vi "mySignInterpreter.vi"() -> ()   [LabVIEW 2017]
uses:
  LeapMotion/TypeDefs/SelectSign.ctl
  LeapMotion/TypeDefs/StateSelector.ctl
  LeapMotion/TypeDefs/AppData.ctl
  MachineLearning/TypeDefs/Label Setting.ctl
  C:/Users/Sara/Documents/GitHub/LEAP-sign-language/LEAP-sign-language/LeapMotion/Dynamic Libraries/LeapCSharp.NET4.5.dll
  LeapMotion/Dynamic Libraries/LeapCSharp.NET4.5.dll
  LeapMotion/LeapMotion.lvlib
  MachineLearning/MachineLearning.lvlib
panel:
  out "Hand count":i32
  in  "Clear text":bool
  in  "Interpret hand sign":bool
  out "Interpreted text":string
  in  "Tab Control":T1(tab)
  out "Real-time plot":cluster{sgl[], sgl[]}[](graph)
  out "Correct interpretations":i32
  out "Number of tries":i32
  out "feature trend":dbl[][](graph)
  out "predicted result":i32[][](graph)
  in  "Error In":errorcluster
  out "Error out":errorcluster
  in  "Trained ML model":path=path "C:/Users/Sara/Documents/GitHub/LEAP-sign-language/LEAP-sign-language/MachineLearning/SubVIs/Models/ASL-ABCD.json"
  out "Accuracy":dbl
  out "Detected sign":T2
  out "Logging in":i32
  in  "Delay":i32=3
  in  "Train model":bool
  out "Points to log":i32
  in  "Start logging":bool
  in  "Write header":bool
  in  "Points/sign":i32=100
  out "feature trend":dbl[][](graph)
  in  "Hand sign":T2
  in  "Stop Program":bool
  out "LEAP connected?":bool
  # "1"
  # "2"
  # "3"
  # "Logging sequence options"
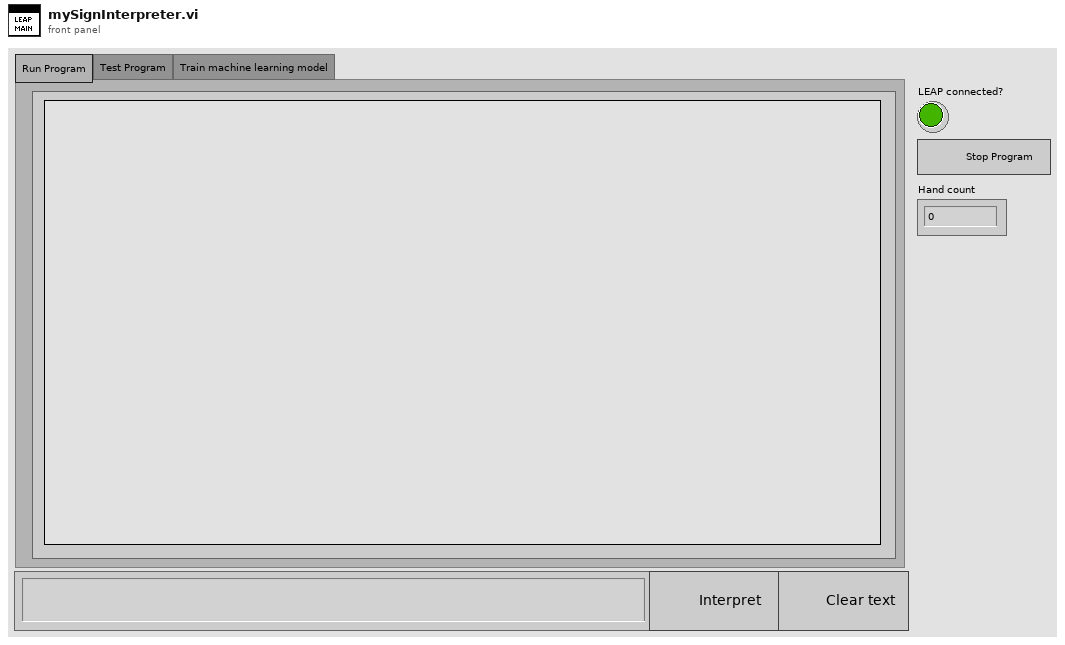
[diagram p1: front panel]
types:
  T1 = enum32{"Run Program", "Test Program", "Train machine learning model"}
  T2 = typedef "LeapMotion.lvlib/SelectSign.ctl" = enum16{"A", "B", "C", "D", "E", "F", "G", "H", "I", "J", "K", "L", "M", "N", "O", "P", "Q", "R", "S", "T", "U", "V", "W", "X", "Y", "Z"}
  T3 = typedef "LeapMotion.lvlib/AppData.ctl" = cluster{"File path":path, "LEAP":refnum<k24>}
  T4 = typedef "LeapMotion.lvlib/StateSelector.ctl" = enum16{"Initialize", "Display", "Write Header", "Logging", "Log gesture", "Train model", "Classify", "Stop"}
  T5 = typedef "MachineLearning.lvlib/Label Setting.ctl" = cluster{"with label column?":bool, "label column index":i32}
  T6 = typedef "LeapMotion.lvlib/LEAPframe.ctl" = cluster{"Id":i64, "Timestamp":i64, "CurrentFramesPerSecond":sgl, "Hands":T7[]}
  T7 = typedef "LeapMotion.lvlib/LEAPhand.ctl" = cluster{"IsLeft":bool, "IsRight":bool, "Id":i32, "FrameId":i64, "Confidence":sgl, "TimeVisible":sgl, "Arm":T8, "PalmPosition":T9, "Fingers":T10[]}
  T8 = typedef "LeapMotion.lvlib/LEAParm.ctl" = cluster{"WristXYZ":sgl[], "CenterXYZ":sgl[], "ElbowXYZ":sgl[]}
  T9 = typedef "LeapMotion.lvlib/LEAPvector.ctl" = cluster{"Pitch":sgl, "Yaw":sgl, "Roll":sgl, "Magnitude":sgl, "XYZ":sgl[]}
  T10 = typedef "LeapMotion.lvlib/LEAPfinger.ctl" = cluster{"IsExtended":bool, "Id":i32, "Type":i32, "HandId":i32, "Length":sgl, "Width":sgl, "TimeVisible":sgl, "TipPosition":T9, "TipVelocity":T9, "Bones":T11[]}
  T11 = typedef "LeapMotion.lvlib/LEAPbone.ctl" = cluster{"Type":i32, "Width":sgl, "Length":sgl, "Center":T9, "Direction":T9, "NextJoint":T9, "PrevJoint":T9}
  T12 = enum16{"SVM", "Neural Network", "Logistic Regression"}
  T13 = cluster{"accuracy":dbl, "precision":dbl, "recall":dbl, "f1 score":dbl}
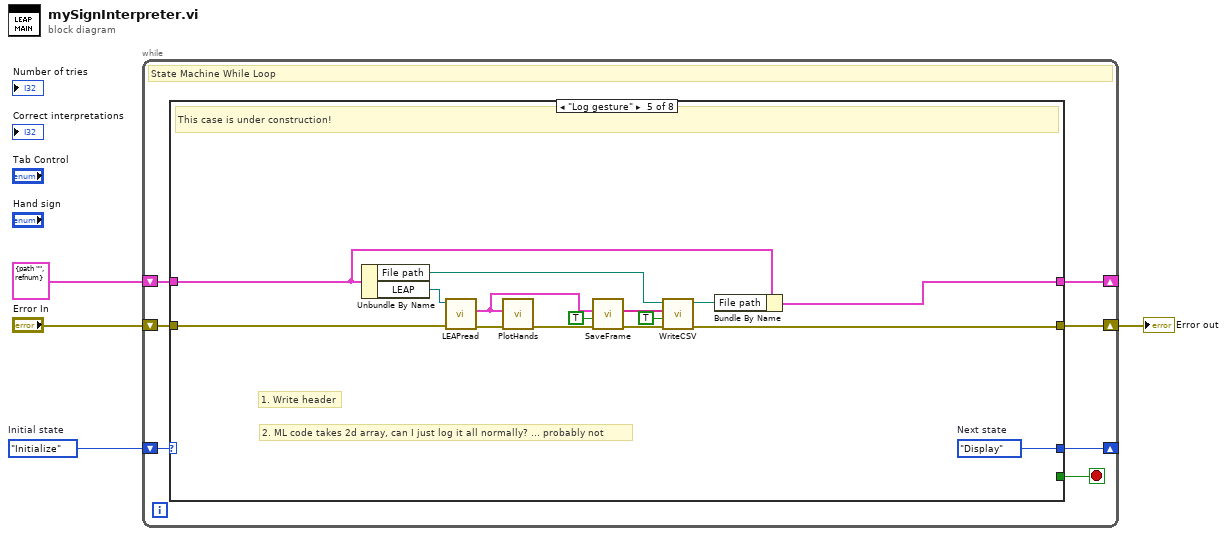
[diagram p0: block diagram]
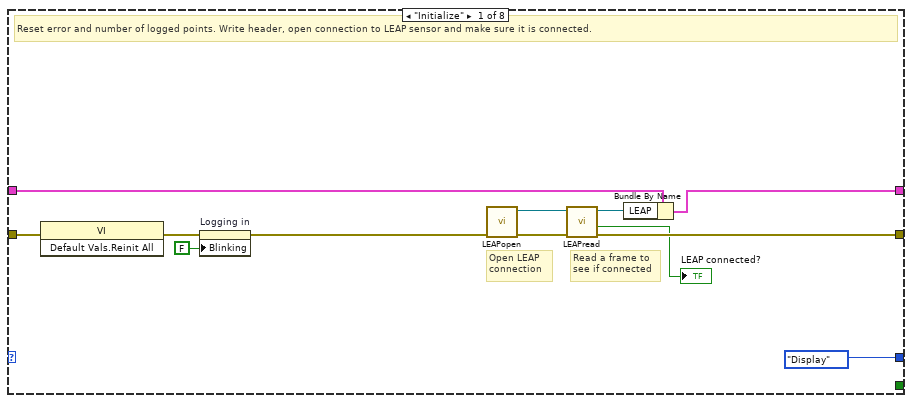
[diagram p2: hidden frame]
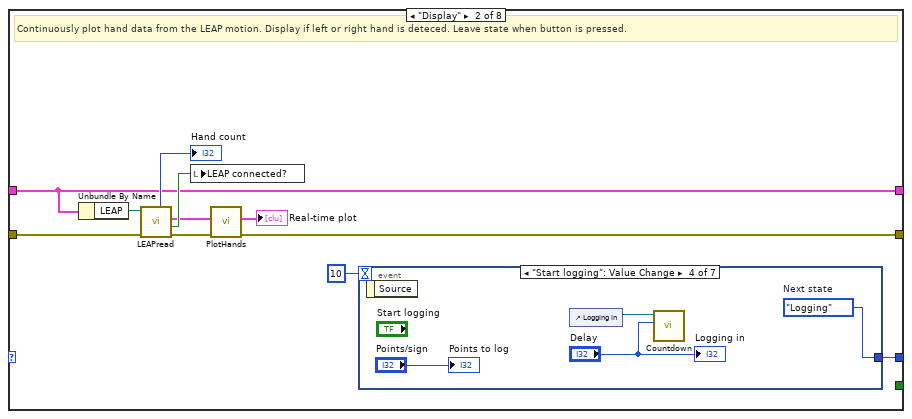
[diagram p3: hidden frame]
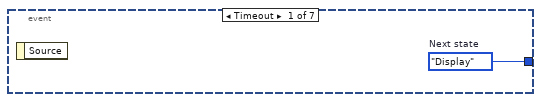
[diagram p4: hidden frame]
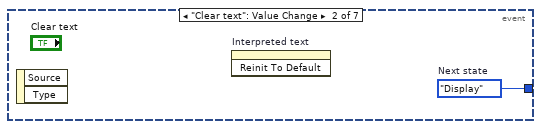
[diagram p5: hidden frame]
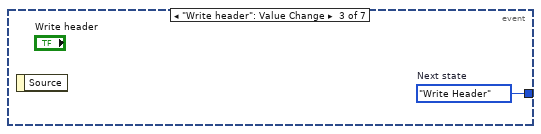
[diagram p6: hidden frame]
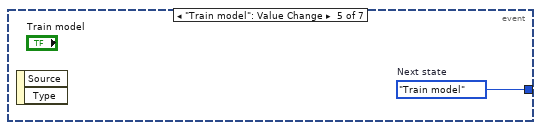
[diagram p7: hidden frame]
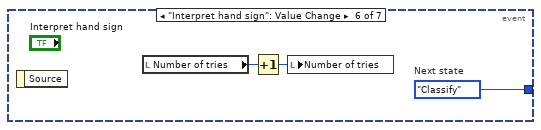
[diagram p8: hidden frame]
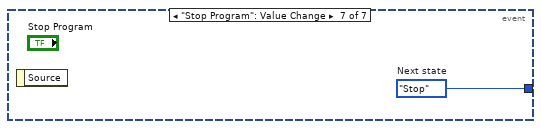
[diagram p9: hidden frame]
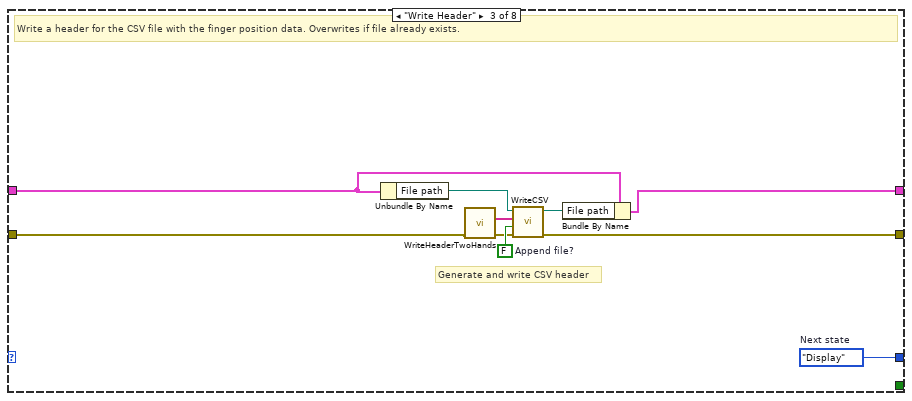
[diagram p10: hidden frame]
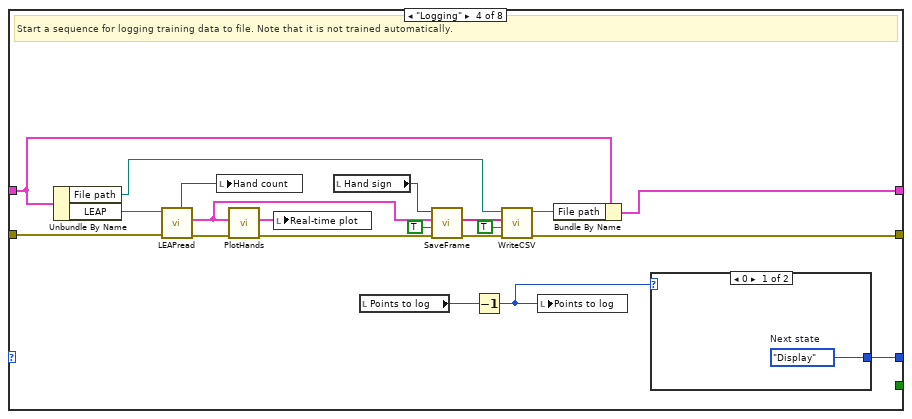
[diagram p11: hidden frame]
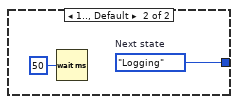
[diagram p12: hidden frame]
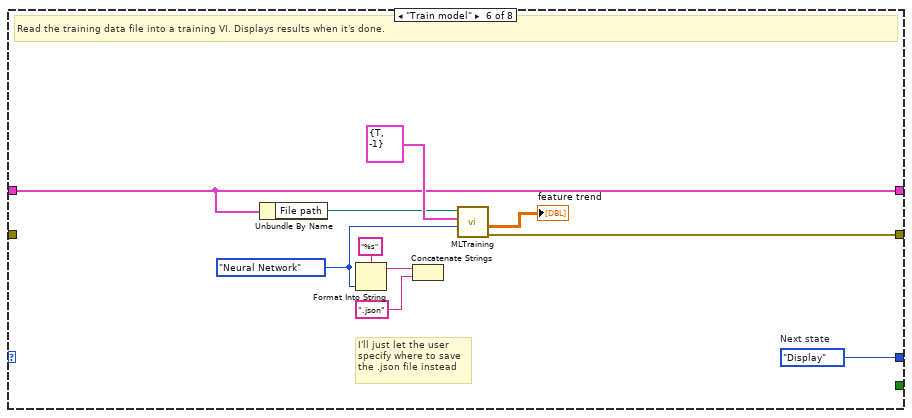
[diagram p13: hidden frame]
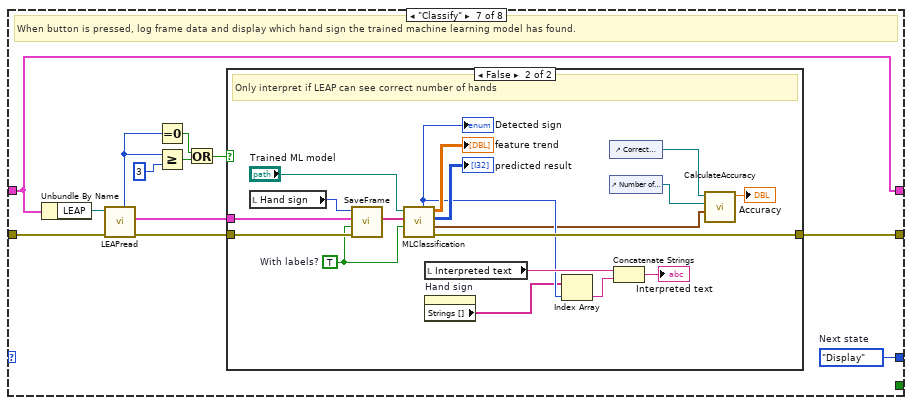
[diagram p14: hidden frame]
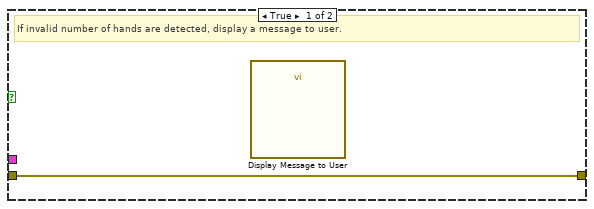
[diagram p15: hidden frame]
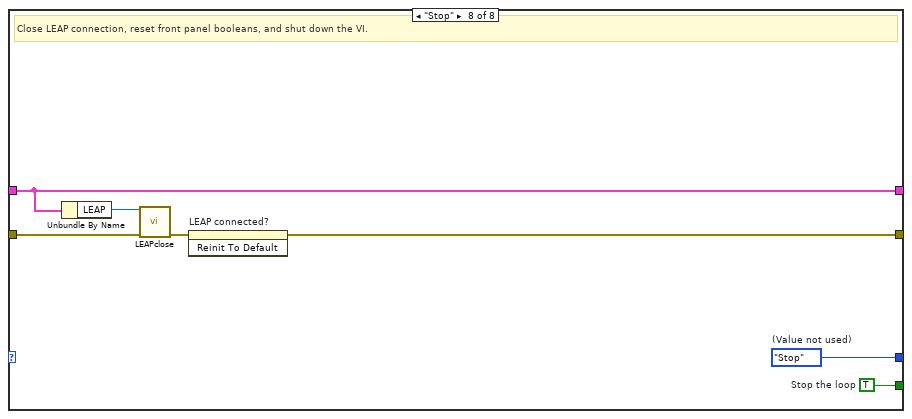
[diagram p16: hidden frame]
diagram:
  w2 = StateSelector."Initialize"  # Initial state
  n1 = while {
    shift-right: [w11] -> w3
    shift-left: "Error In" -> [w10]
    shift-right: [w8] -> _
    shift-left: w2 -> [w5]
    shift-right: [w6] -> _
    shift-left: T3 {"File path"=path "", "LEAP"=refnum} -> [w7]
    stop <- w9 stop-if-true
    # "State Machine While Loop"
    n2 = case "State Machine Case Structure" shown="\"Log gesture\"" w5 {
      tunnel: [_ _ _ _ _ _ _ w142] -> w9
      tunnel: [w20 w31 w56 w69 w82 w104 w113 w136] -> w11
      tunnel: w10 -> [w23 w33 w51 w76 w83 _ w116 w141]
      tunnel: [StateSelector."Display" ("Enum") w29 w54 w67 w94 w98 w112 w139] -> w8
      tunnel: w7 -> [w15 w26 w50 w60 w84 w96 w105 w137]
      tunnel: [w13 w26 w49 w63 w81 w96 w105 w137] -> w6
      frame "Initialize" {
        # "Read a frame to\nsee if connected"
        # "Open LEAP \nconnection"
        # "Reset error and number of logged points. Write header, open connection to LEAP sensor and make sure it is connected."
        n3 = invoke class="VI" method="Default Vals.Reinit All"(error in=w23) -> (error out=w17:errorcluster)  [unwired: 2 in, 2 out]
        n4 = property on="Logging in" class="DigNum (strict)"(error in=w17, "Blinking"=FALSE) -> (error out=w16:errorcluster)  [unwired: 1 in, 1 out]
        n5 = call "LEAPopen.vi"("error in (no error)"=w16) -> ("error out"=w21:errorcluster, "Leap.Controller"=w22:refnum<k24>)  [unwired: 9 in]
        n6 = call "LEAPread.vi"("error in (no error)"=w21, "Controller Refnum In"=w22) -> ("error out"=w20:errorcluster, "IsConnected"=→"LEAP connected?":bool, "Leap.Controller"=w14:refnum<k24>)  [unwired: 5 in, 2 out]
        n7 = Bundle By Name(cluster=w15, "LEAP"=w14) -> (w13:T3)
      }
      frame "Display" {
        # "Continuously plot hand data from the LEAP motion. Display if left or right hand is deteced. Leave state when button is pressed."
        n8 = Unbundle By Name(w26) -> ("LEAP"=w27:refnum<k24>)
        n9 = call "LEAPread.vi"("error in (no error)"=w33, "Controller Refnum In"=w27) -> ("error out"=w30:errorcluster, "IsConnected"=w32:bool, "Frame"=w25:T6, "Hand count"=→"Hand count":i32)  [unwired: 5 in, 1 out]
        n10 = local write "LEAP connected?"(w32) -> ()
        n11 = call "PlotHands.vi"("error in"=w30, "Frame"=w25) -> ("error out"=w31:errorcluster, "Data to plot"=→"Real-time plot":cluster{"Array":sgl[], "Array":sgl[]}[])  [unwired: 8 in]
        n12 = event shown="[3] \"Start logging\": Value Change" {
          selector: _ -> [_ _ _ _ _ _ _]
          dyn-events: _ -> [_ _ _ _ _ _ _]
          timeout: 10 -> [_ _ _ _ _ _ _]
          tunnel: [w35 w36 w37 w41 w42 w45 w46] -> w29
          event Timeout {
            w35 = StateSelector."Display"  # Next state
            n13 = event-data() -> ()  [unwired: 1 in, 1 out]
          }
          event "Clear text": Value Change {
            w36 = StateSelector."Display"  # Next state
            n14 = event-data() -> ()  [unwired: 1 in, 2 out]
            n15 = invoke on="Interpreted text" class="Str" method="Reinit To Default"() -> ()  [unwired: 3 in, 3 out]
          }
          event "Write header": Value Change {
            w37 = StateSelector."Write Header"  # Next state
            n16 = event-data() -> ()  [unwired: 1 in, 1 out]
          }
          event "Start logging": Value Change {
            w41 = StateSelector."Logging"  # Next state
            n17 = event-data() -> ()  [unwired: 1 in, 1 out]
            n18 = control-ref of="Logging in"() -> (w38:refnum<vi>)
            n19 = call "Countdown.vi"("Delay before logging"="Delay", "Digital in"=w38) -> ()  [unwired: 10 in]
            "Points to log" <- "Points/sign"
            "Logging in" <- "Delay"
          }
          event "Train model": Value Change {
            w42 = StateSelector."Train model"  # Next state
            n20 = event-data() -> ()  [unwired: 1 in, 2 out]
          }
          event "Interpret hand sign": Value Change {
            w45 = StateSelector."Classify"  # Next state
            n21 = event-data() -> ()  [unwired: 1 in, 1 out]
            n22 = local read "Number of tries"() -> (w44:i32)
            n23 = Increment(x=w44) -> (x+1=w43:i32)
            n24 = local write "Number of tries"(w43) -> ()
          }
          event "Stop Program": Value Change {
            w46 = StateSelector."Stop"  # Next state
            n25 = event-data() -> ()  [unwired: 1 in, 1 out]
          }
        }
      }
      frame "Write Header" {
        w55 = FALSE  # Append file?
        w54 = StateSelector."Display"  # Next state
        # "Generate and write CSV header"
        # "Write a header for the CSV file with the finger position data. Overwrites if file already exists."
        n26 = Unbundle By Name(w50) -> ("File path"=w48:path)
        n27 = call "WriteHeaderTwoHands.vi"("Error in"=w51) -> ("Error out"=w52:errorcluster, "Header string array"=w53:string[])  [unwired: 9 in]
        n28 = call "WriteCSV.vi"("error in (no error)"=w52, "Append file?"=w55, "Data to write"=w53, "CSV file path in"=w48) -> ("error out"=w56:errorcluster, "CSV file path out"=w47:path)  [unwired: 6 in]
        n29 = Bundle By Name(cluster=w50, "File path"=w47) -> (w49:T3)
      }
      frame "Logging" {
        # "Start a sequence for logging training data to file. Note that it is not trained automatically."
        n30 = Unbundle By Name(w60) -> ("File path"=w59:path, "LEAP"=w61:refnum<k24>)
        n31 = call "LEAPread.vi"("error in (no error)"=w76, "Controller Refnum In"=w61) -> ("error out"=w66:errorcluster, "Frame"=w58:T6, "Hand count"=w64:i32)  [unwired: 5 in, 2 out]
        n32 = local write "Hand count"(w64) -> ()
        n33 = call "PlotHands.vi"("error in"=w66, "Frame"=w58) -> ("error out"=w65:errorcluster, "Data to plot"=w57:cluster{"Array":sgl[], "Array":sgl[]}[])  [unwired: 8 in]
        n34 = local write "Real-time plot"(w57) -> ()
        n35 = local read "Hand sign"() -> (w74:T2)
        n36 = local read "Points to log"() -> (w71:i32)
        n37 = call "SaveFrame.vi"("Error In"=w65, "With labels?"=TRUE, "Frame"=w58, "Hand sign"=w74) -> ("Error Out"=w75:errorcluster, "Frame data"=w73:string[])  [unwired: 6 in]
        n38 = Decrement(x=w71) -> (x-1=w68:i32)
        n39 = call "WriteCSV.vi"("error in (no error)"=w75, "Append file?"=TRUE, "Data to write"=w73, "CSV file path in"=w59) -> ("error out"=w69:errorcluster, "CSV file path out"=w62:path)  [unwired: 6 in]
        n40 = local write "Points to log"(w68) -> ()
        n41 = Bundle By Name(cluster=w60, "File path"=w62) -> (w63:T3)
        n42 = case shown="0" w68 {
          tunnel: [w77 w79] -> w67
          frame 0 {
            w77 = StateSelector."Display"  # Next state
          }
          frame 1.., Default {
            w79 = StateSelector."Logging"  # Next state
            n43 = Wait (ms)(milliseconds to wait=u32 50) -> ()  [unwired: 1 out]
          }
        }
      }
      frame "Log gesture" {
        w94 = StateSelector."Display"  # Next state
        # "2. ML code takes 2d array, can I just log it all normally? ... probably not"
        # "1. Write header"
        # "This case is under construction!"
        n44 = Unbundle By Name(w84) -> ("File path"=w85:path, "LEAP"=w86:refnum<k24>)
        n45 = call "LEAPread.vi"("error in (no error)"=w83, "Controller Refnum In"=w86) -> ("error out"=w89:errorcluster, "Frame"=w80:T6)  [unwired: 5 in, 3 out]
        n46 = call "PlotHands.vi"("error in"=w89, "Frame"=w80) -> ("error out"=w88:errorcluster)  [unwired: 8 in, 1 out]
        n47 = call "SaveFrame.vi"("Error In"=w88, "With labels?"=TRUE, "Frame"=w80) -> ("Error Out"=w93:errorcluster, "Frame data"=w92:string[])  [unwired: 7 in]
        n48 = call "WriteCSV.vi"("error in (no error)"=w93, "Append file?"=TRUE, "Data to write"=w92, "CSV file path in"=w85) -> ("error out"=w82:errorcluster, "CSV file path out"=w87:path)  [unwired: 6 in]
        n49 = Bundle By Name(cluster=w84, "File path"=w87) -> (w81:T3)
      }
      frame "Train model" {
        w101 = T12."Neural Network" ("model to train")
        w98 = StateSelector."Display"  # Next state
        # "I'll just let the user\nspecify where to save\nthe .json file instead"
        # "Read the training data file into a training VI. Displays results when it's done."
        n50 = Unbundle By Name(w96) -> ("File path"=w95:path)
        n51 = Format Into String(format string="%s", w101) -> (resulting string=w100:string)  [unwired: 2 in, 1 out]
        n52 = Concatenate Strings(w100, ".json" ("string")) -> ()  [unwired: 1 out]
        n53 = call "MLTraining.vi"("model to train"=w101, "Label setting"=T5 {"with label column?"=TRUE, "label column index"=-1}, "training data file (CSV)"=w95) -> ("error out"=w104:errorcluster, "feature trend"=→"feature trend":dbl[][])  [unwired: 7 in]
      }
      frame "Classify" {
        w112 = StateSelector."Display"  # Next state
        # "When button is pressed, log frame data and display which hand sign the trained machine learning model has found."
        n54 = Unbundle By Name(w105) -> ("LEAP"=w106:refnum<k24>)
        n55 = call "LEAPread.vi"("error in (no error)"=w116, "Controller Refnum In"=w106) -> ("error out"=w115:errorcluster, "Frame"=w114:T6, "Hand count"=w107:i32)  [unwired: 5 in, 2 out]
        n56 = Equal To 0?(x=w107) -> (x = 0?=w109:bool)
        n57 = Greater Or Equal?(x=w107, y=3) -> (x >= y?=w108:bool)
        n58 = Or(x=w109, y=w108) -> (x .or. y?=w110:bool)
        n59 = case shown="False" w110 {
          tunnel: w115 -> [w117 w132]
          tunnel: w114 -> [_ w131]
          tunnel: [w117 w128] -> w113
          frame True {
            # "If invalid number of hands are detected, display a message to user."
            n60 = call "Display Message to User"() -> ()  [unwired: 10 in, 2 out]
          }
          frame False {
            w124 = TRUE  # With labels?
            # "Only interpret if LEAP can see correct number of hands"
            n61 = local read "Hand sign"() -> (w125:T2)
            n62 = call "SaveFrame.vi"("Error In"=w132, "With labels?"=w124, "Frame"=w131, "Hand sign"=w125) -> ("Frame data"=w123:string[])  [unwired: 6 in, 1 out]
            n63 = call "MLClassification.vi"("with labels?"=w124, "Frame data"=w123, "model file (JSON)"="Trained ML model") -> ("error out"=w128:errorcluster, "metrics"=w121:T13, "predicted result"=→"predicted result":i32[][], "feature trend"=→"feature trend":dbl[][], "Detected hand sign"=w126:i32)  [unwired: 4 in]
            "Detected sign" <- w126
            n64 = local read "Interpreted text"() -> (w135:string)
            n65 = property on="Hand sign" class="Enum (strict)"() -> ("Strings []"=w122:string[])  [unwired: 2 in, 2 out]
            n66 = Index Array(array=w122, index=w126) -> (element=w133:string)
            n67 = control-ref of="Correct interpretations"() -> (w119:refnum<vi>)
            n68 = control-ref of="Number of tries"() -> (w120:refnum<vi>)
            n69 = Concatenate Strings(w135, w133) -> (→"Interpreted text":string)
            n70 = call "CalculateAccuracy.vi"("metrics"=w121, "Number of tries"=w120, "Correct interpretations"=w119) -> ("Accuracy"=→"Accuracy":dbl)  [unwired: 8 in]
          }
        }
      }
      frame "Stop" {
        w142 = TRUE  # Stop the loop
        w139 = StateSelector."Stop"  # (Value not used)
        # "Close LEAP connection, reset front panel booleans, and shut down the VI."
        n71 = Unbundle By Name(w137) -> ("LEAP"=w138:refnum<k24>)
        n72 = call "LEAPclose.vi"("error in (no error)"=w141, ".NET Refnum in"=w138) -> ("error out"=w140:errorcluster)  [unwired: 9 in]
        n73 = invoke on="LEAP connected?" class="Bool (strict)" method="Reinit To Default"(error in=w140) -> (error out=w136:errorcluster)  [unwired: 2 in, 2 out]
      }
    }
  }
  "Error out" <- w3
